vi "Untitled 12.vi"() -> ()   [LabVIEW 2010]
uses:
  <vilib>/NXT/Block Support/NXT_InputPort.ctl
  <vilib>/NXT/Subs/MotorOutput.ctl
  <vilib>/NXT/Dual Mode Library/Sensors/Light_On.vi
  <vilib>/NXT/Dual Mode Library/Motors/MotorOn.vi
  <vilib>/NXT/Dual Mode Library/Waits/Wait_Num.vi
  <vilib>/NXT/Dual Mode Library/Motors/MotorReverse.vi
panel:
  in  "Output Port (All Ports)":T1=3 items=["Port A", "Port B", "Port C", "All Ports"]
  in  "stop":bool
  in  "파워":i32=75
  in  "오른쪽 모터":T1=3 items=["Port A", "Port B", "Port C", "All Ports"]
  in  "왼쪽 모터":T1=3 items=["Port A", "Port B", "Port C", "All Ports"]
  in  "빛센서":T2=2 items=["Port 1", "Port 2", "Port 3", "Port 4"]
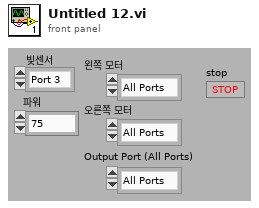
[diagram p1: front panel]
types:
  T1 = typedef "MotorOutput.ctl" = u8
  T2 = typedef "NXT_InputPort.ctl" = u8
  T3 = typedef "LVHSConnector.ctl" = cluster{"error":errorcluster, "address":string, "NXT #":i32, "Show Error":bool, "Connection":u16}
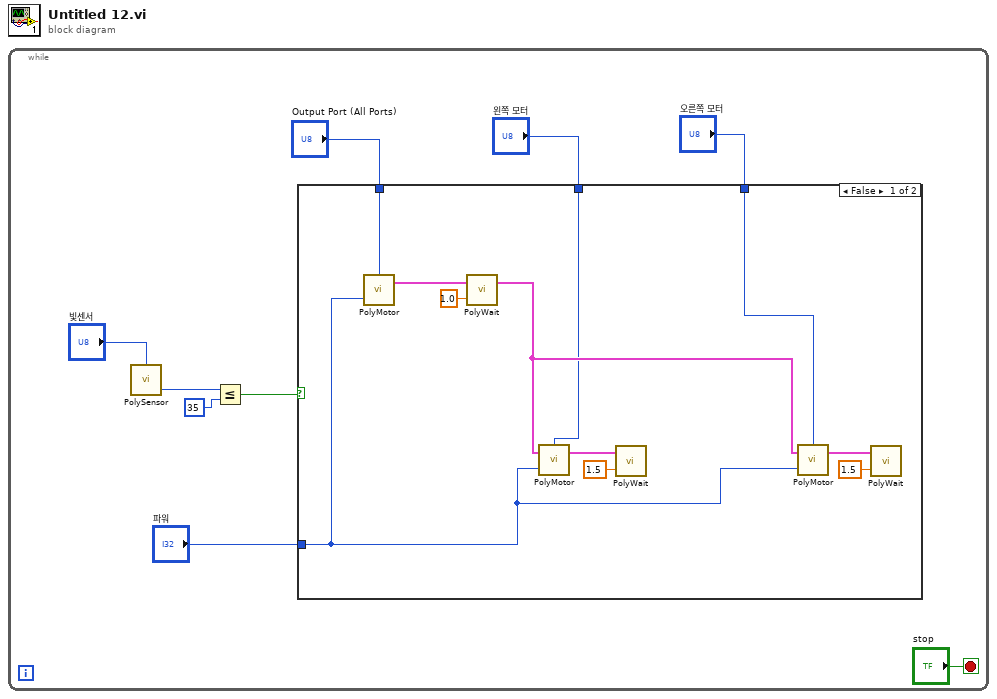
[diagram p0: block diagram]
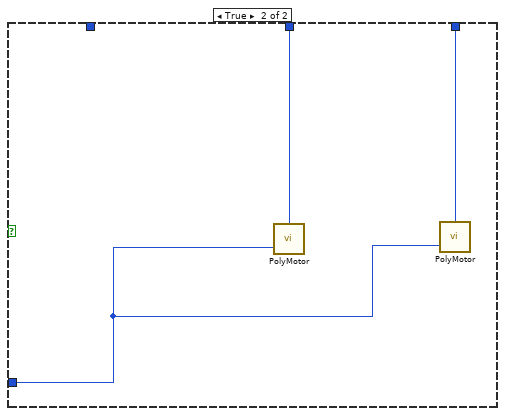
[diagram p2: hidden frame]
diagram:
  n1 = while {
    stop <- "stop" stop-if-true
    n2 = call-poly <vilib>:"PolySensor.vi"("Port (Port 3)"="빛센서") -> ("Scaled Value"=w1:i16)  [unwired: 2 in, 1 out]
    n3 = Less Or Equal?(x=w1, y=i16 35) -> (x <= y?=w2:bool)
    n4 = case shown="False" w2 {
      tunnel: "오른쪽 모터" -> [w15 w23]
      tunnel: "왼쪽 모터" -> [w16 w22]
      tunnel: "파워" -> [w10 w21]
      tunnel: "Output Port (All Ports)" -> [w18 _]
      frame False {
        n5 = call-poly <vilib>:"PolyMotor.vi"("Power (75)"=w10, "Output Port (All Ports)"=w18) -> ("NXT"=w19:T3)  [unwired: 2 in]
        n6 = call-poly <vilib>:"PolyWait.vi"("Time (sec)"=sgl 1.0, "NXT"=w19) -> ("NXT"=w17:T3)  [unwired: 2 in]
        n7 = call-poly <vilib>:"PolyMotor.vi"("Power (75)"=w10, "NXT"=w17, "Output Port (All Ports)"=w16) -> ("NXT"=w14:T3)  [unwired: 1 in]
        n8 = call-poly <vilib>:"PolyWait.vi"("Time (sec)"=sgl 1.5, "NXT"=w14) -> ()  [unwired: 2 in, 1 out]
        n9 = call-poly <vilib>:"PolyMotor.vi"("Power (75)"=w10, "NXT"=w17, "Output Port (All Ports)"=w15) -> ("NXT"=w13:T3)  [unwired: 1 in]
        n10 = call-poly <vilib>:"PolyWait.vi"("Time (sec)"=sgl 1.5, "NXT"=w13) -> ()  [unwired: 2 in, 1 out]
      }
      frame True {
        n11 = call-poly <vilib>:"PolyMotor.vi"("Power (75)"=w21, "Output Port (All Ports)"=w22) -> ()  [unwired: 2 in, 1 out]
        n12 = call-poly <vilib>:"PolyMotor.vi"("Power (75)"=w21, "Output Port (All Ports)"=w23) -> ()  [unwired: 2 in, 1 out]
      }
    }
  }
